vi "From LabVIEW.vi"(4 "AlbumMap in":refnum<class "AlbumMap.lvclass">, 8 "error in (no error)":errorcluster, 10 "Value":refnum<class>) -> (0 "error out":errorcluster, 2 "DbRow":variant)   [LabVIEW 2020, in "ORM_Examples.lvlib" / "AlbumMap.lvclass"]
uses:
  AlbumMap.lvclass
  C:/Program Files/National Instruments/LabVIEW 2024/vi.lib/Viviota/shared/ORM.lvlibp/ORM/TypeMap/TypeMap.lvclass
  Album/Album.lvclass
  Album/Album.lvclass/Album.ctl
  Album/Read Title.vi
  Album/Read Primary Key.vi
  <vilib>/Viviota/shared/ORM.lvlibp/ORM/TypeMap/Read Autokey.vi
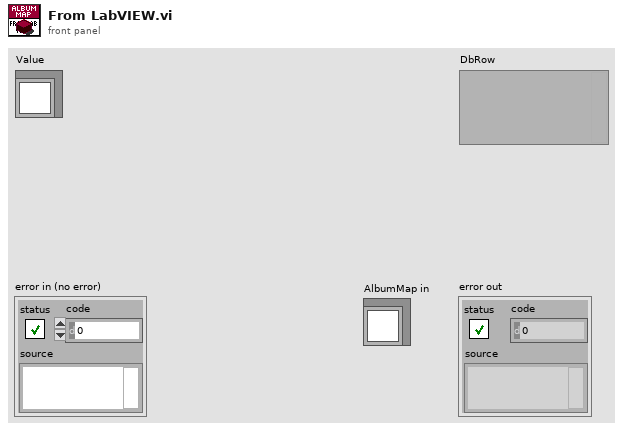
[diagram p1: front panel]
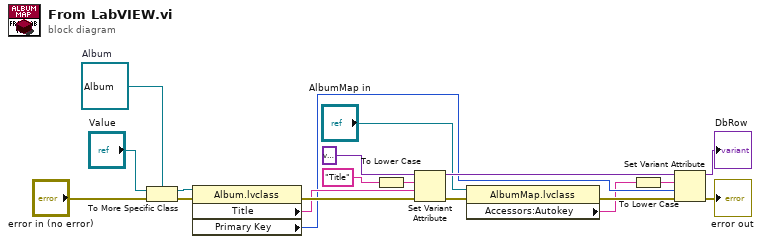
[diagram p0: block diagram]
diagram:
  w12 = refnum<class "Album.lvclass"> refnum  # Album
  n1 = To More Specific Class(target class=w12, reference="Value", error in="error in (no error)") -> (specific class reference=w11:refnum<class "Album.lvclass">, error out=w10:errorcluster)
  n2 = property class="Album.lvclass"(reference=w11, error in=w10) -> (error out=w16:errorcluster, "Title"=w15:string, "Primary Key"=w9:i64)  [unwired: 1 out]
  n3 = To Lower Case(string="Title" ("name")) -> (all lower case string=w1:string)
  n4 = Set Variant Attribute(Variant=variant, name=w1, value=w15, error in=w16) -> (Variant out=w19:variant, error out=w17:errorcluster)  [unwired: 1 out]
  n5 = property class="AlbumMap.lvclass"(reference="AlbumMap in", error in=w17) -> (error out=w18:errorcluster, "Accessors:Autokey"=w7:string)  [unwired: 1 out]
  n6 = To Lower Case(string=w7) -> (all lower case string=w2:string)
  n7 = Set Variant Attribute(Variant=w19, name=w2, value=w9, error in=w18) -> (Variant out=→"DbRow":variant, error out=→"error out":errorcluster)  [unwired: 1 out]
